vi "Reset Control.vi"(0 "GEA2 Reference In":refnum<k24>, 11 "Error In":errorcluster) -> (4 "GEA2 Reference Out":refnum<k24>, 6 "Pass/Fail?":bool, 8 "Report Text":string, 15 "Error Out":errorcluster)   [LabVIEW 2016, in "Centauro.lvlib"]
doc: "Use this VI to reset the board."
uses:
  Projects/Centauro.lvlib
  Q:/Common/DLLs/GEA3/GeaCommunication.dll
  Common/DLLs/GEA3/GeaCommunication.dll
  Common/LabVIEW GEA2 Toolkit/LabVIEW_GEA2_Toolkit.lvlibp/type defs/ERD Write Data In.ctl
  Common/LabVIEW GEA2 Toolkit/LabVIEW_GEA2_Toolkit.lvlibp/type defs/Data Type.ctl
  Common/LabVIEW GEA2 Toolkit/LabVIEW_GEA2_Toolkit.lvlibp/type defs/Source_Destination.ctl
  Common/LabVIEW GEA2 Toolkit/LabVIEW_GEA2_Toolkit.lvlibp
panel:
  out "Time to fault code clear":dbl
  out "Time to fault code set (s)":dbl
  in  "Standalone?":bool
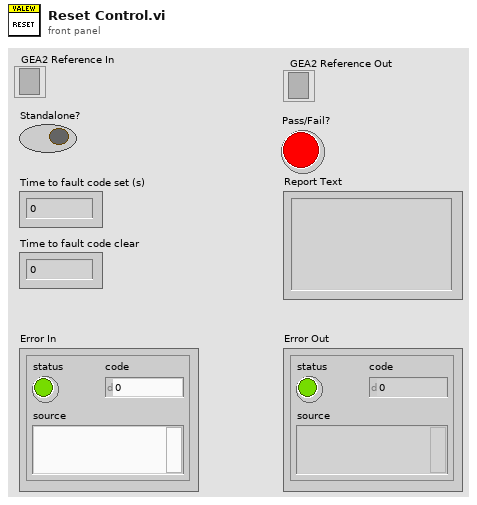
[diagram p1: front panel]
types:
  T1 = typedef "LabVIEW_GEA2_Toolkit.lvlibp/ERD Write Data In.ctl" = cluster{"ERD Number":u16, "Data Type":T2, "Data":string}
  T2 = typedef "LabVIEW_GEA2_Toolkit.lvlibp/Data Type.ctl" = enum16{"string", "boolean", "uint8_t", "uint16_t", "uint32_t", "uint64_t", "int8_t", "int16_t", "int32_t", "int64_t"}
  T3 = typedef "LabVIEW_GEA2_Toolkit.lvlibp/Source_Destination.ctl" = cluster{"Source":u8, "Destination":u8}
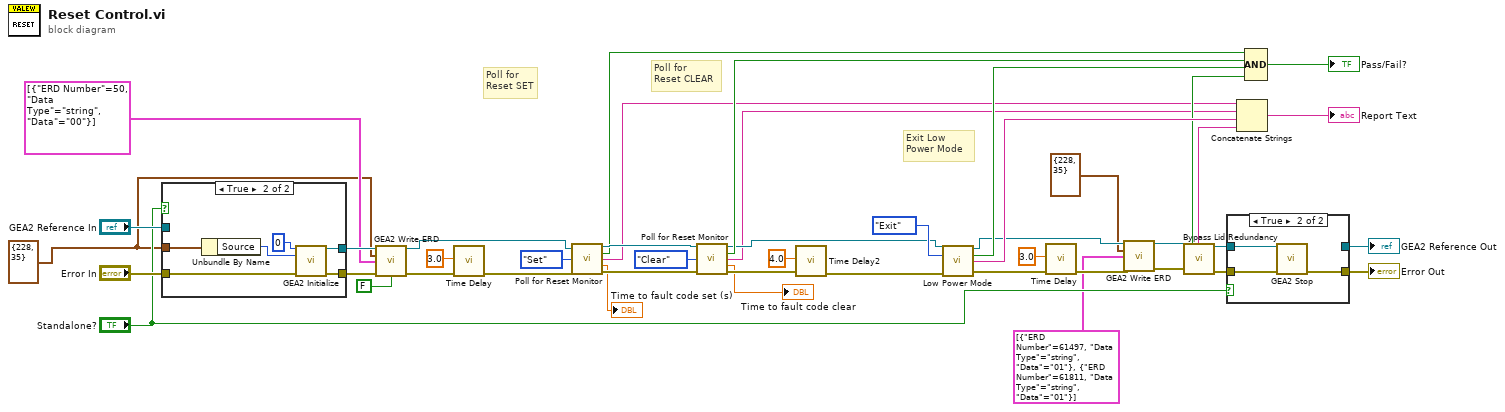
[diagram p0: block diagram]
diagram:
  w21 = T3 {"Source"=228, "Destination"=35} ("GEA Inputs")
  # "Exit Low \nPower Mode"
  # "Poll for\nReset CLEAR"
  # "Poll for\nReset SET"
  n1 = case shown="True" "Standalone?" {
    tunnel: "Error In" -> [w46 w53]
    tunnel: [w46 w52] -> w40
    tunnel: "GEA2 Reference In" -> [w47 _]
    tunnel: [w47 w51] -> w45
    tunnel: w21 -> [_ w49]
    frame False {
    }
    frame True {
      n2 = Unbundle By Name(w49) -> ("Source"=w50:u8)
      n3 = call "GEA2 Initialize.vi"("Board Index"=0, "Source Address"=w50, "error in"=w53) -> ("GEA2 Reference Out"=w51:refnum<k24>, "error out"=w52:errorcluster)  [unwired: 10 in, 1 out]
    }
  }
  n4 = call "GEA2 Write ERD.vi"("GEA2 Reference In"=w45, "GEA Inputs"=w21, "Write ERD List"=T1[] [{"ERD Number"=50, "Data Type"=enum."string", "Data"="00"}], "Error In"=w40, "Verify ERD Response?"=FALSE) -> ("GEA2 Reference Out"=w16:refnum<k24>, "Error Out"=w32:errorcluster)  [unwired: 8 in, 1 out]
  n5 = call "Time Delay"("error in (no error)"=w32, "Delay Time (s)"=3.0) -> ("error out"=w20:errorcluster)  [unwired: 9 in]
  n6 = call "Poll for Reset Monitor.vi"("GEA2 Reference In"=w16, "Status"=enum16{"Clear", "Set"}."Set", "Error In"=w20) -> ("GEA2 Reference Out"=w15:refnum<k24>, "Pass/Fail?"=w14:bool, "Report Text"=w9:string, "Time until condition met (s)"=→"Time to fault code set (s)":dbl, "Error Out"=w18:errorcluster)  [unwired: 8 in]
  n7 = call "Poll for Reset Monitor.vi"("GEA2 Reference In"=w15, "Status"=enum16{"Clear", "Set"}."Clear", "Error In"=w18) -> ("GEA2 Reference Out"=w12:refnum<k24>, "Pass/Fail?"=w13:bool, "Report Text"=w10:string, "Time until condition met (s)"=→"Time to fault code clear":dbl, "Error Out"=w11:errorcluster)  [unwired: 8 in]
  n8 = call "Time Delay2"("error in (no error)"=w11, "Delay Time (s)"=4.0) -> ("error out"=w26:errorcluster)  [unwired: 9 in]
  n9 = call "Low Power Mode.vi"("GEA2 Reference In"=w12, "Action"=enum16{"Enter", "Exit"}."Exit", "Error In"=w26) -> ("GEA2 Reference Out"=w3:refnum<k24>, "Pass/Fail?"=w34:bool, "Report Text"=w37:string, "Error Out"=w28:errorcluster)  [unwired: 9 in]
  n10 = call "Time Delay"("error in (no error)"=w28, "Delay Time (s)"=3.0) -> ("error out"=w6:errorcluster)  [unwired: 9 in]
  n11 = call "GEA2 Write ERD.vi"("GEA2 Reference In"=w3, "GEA Inputs"=T3 {"Source"=228, "Destination"=35}, "Write ERD List"=T1[] [{"ERD Number"=61497, "Data Type"=enum."string", "Data"="01"}, {"ERD Number"=61811, "Data Type"=enum."string", "Data"="01"}], "Error In"=w6) -> ("GEA2 Reference Out"=w4:refnum<k24>, "Error Out"=w5:errorcluster)  [unwired: 9 in, 1 out]
  n12 = call "Bypass Lid Redundancy.vi"("GEA2 Reference In"=w4, "Error In"=w5) -> ("GEA2 Reference Out"=w24:refnum<k24>, "Pass/Fail?"=w23:bool, "Report Text"=w22:string, "Error Out"=w25:errorcluster)  [unwired: 10 in]
  n13 = case shown="True" "Standalone?" {
    tunnel: w25 -> [w55 w58]
    tunnel: [w55 w57] -> w44
    tunnel: [w54 _] -> w43
    tunnel: w24 -> [w54 w56]
    frame False {
    }
    frame True {
      n14 = call "GEA2 Stop.vi"("GEA2 Reference In"=w56, "Error In"=w58) -> ("Error Out"=w57:errorcluster)  [unwired: 13 in]
    }
  }
  "Error Out" <- w44
  "GEA2 Reference Out" <- w43
  n15 = Concatenate Strings(w9, w10, w37, w22) -> (→"Report Text":string)
  n16 = Compound Arithmetic op=AND(w14, w13, w34, w23) -> (→"Pass/Fail?":bool)
